vi "Communication Manager.vi"(7 "Mode":T1(ring)=enum."Get References", 8 "error in":errorcluster, 9 "Error Queue":refnum<queue>, 11 "Application Events":refnum<user-event>) -> (0 "error out":errorcluster, 1 "Error Queue Out":refnum<queue>, 3 "Application Events Out":refnum<user-event>)   [LabVIEW 2020, in "Error Handler.lvlib"]
doc: "Holds reference to communication structure need by the current module both for internal and external use"
uses:
  Error Handler.lvlib
  Controls/Error Message Object.ctl
  Controller/Controls/Application Modules.ctl
  Controls/Error Commands.ctl
  Controller/Controls/Application Event Object.ctl
  Controller/Controls/Application Events.ctl
  Controller/Controller.lvlib
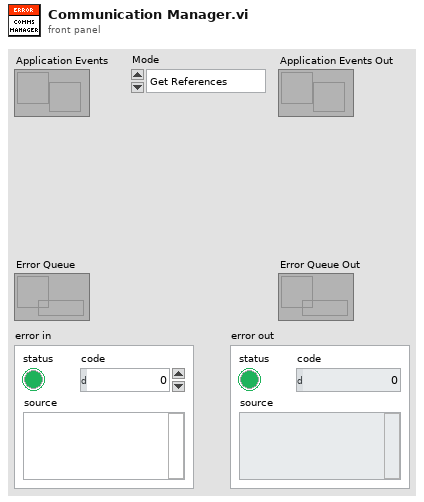
[diagram p1: front panel]
types:
  T1 = enum16{"Load References", "Release References", "Get References"}
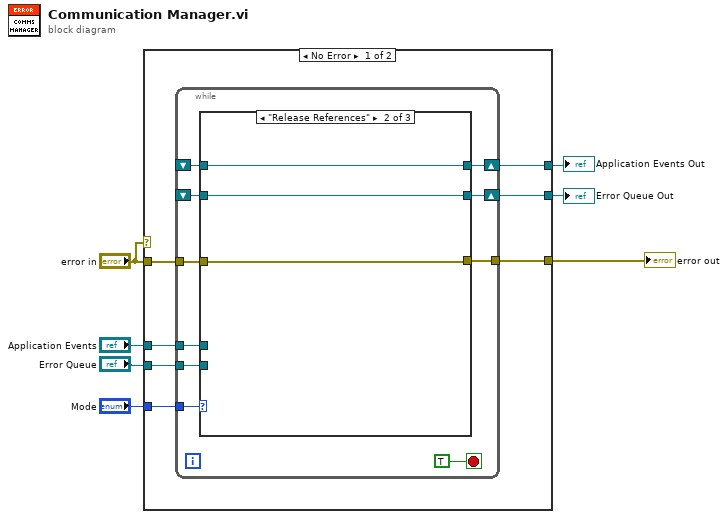
[diagram p0: block diagram]
diagram:
  n1 = case shown="No Error" "error in" {
    tunnel: [w11 w34] -> w7
    tunnel: "error in" -> [w12 w34]
    tunnel: "Application Events" -> [w14 _]
    tunnel: "Error Queue" -> [w13 _]
    tunnel: [w10 _] -> w3
    tunnel: [w9 _] -> w2
    tunnel: "Mode" -> [w8 _]
    frame No Error {
      n2 = while {
        tunnel: w14 -> [w22]
        shift-right: [w23] -> w10
        shift-left: _ -> [w21]
        shift-right: [w20] -> w9
        shift-left: _ -> [w19]
        tunnel: w13 -> [w18]
        tunnel: w12 -> [w17]
        tunnel: [w16] -> w11
        tunnel: w8 -> [w15]
        stop <- TRUE stop-if-true
        n3 = case shown="\"Release References\"" w15 {
          tunnel: [w26 w30 w33] -> w23
          tunnel: w22 -> [_ _ w33]
          tunnel: w21 -> [w26 w30 _]
          tunnel: [w25 w29 w32] -> w20
          tunnel: w19 -> [w25 w29 _]
          tunnel: w18 -> [_ _ w32]
          tunnel: w17 -> [w27 w28 w31]
          tunnel: [w27 w28 w31] -> w16
          frame Default {
          }
          frame "Release References" {
          }
          frame "Load References" {
          }
        }
      }
    }
    frame Error {
    }
  }
  "error out" <- w7
  "Application Events Out" <- w3
  "Error Queue Out" <- w2
